vi "Lire Parameters.vi"(11 "Operation en entrée":refnum<class "Operation.lvclass">) -> (2 "Parameters":T1 {"Currency" items=["Euro", "Dollar", "Yen", "RIM", "CHF"]}, 3 "Operation en sortie":refnum<class "Operation.lvclass">)   [LabVIEW 2012, in "Operation.lvclass"]
uses:
  Operation.lvclass
  Operation Parameters.ctl
  Operation Type Enum.ctl
  controls/Currencies.ctl
  Operation.lvclass/Operation.ctl
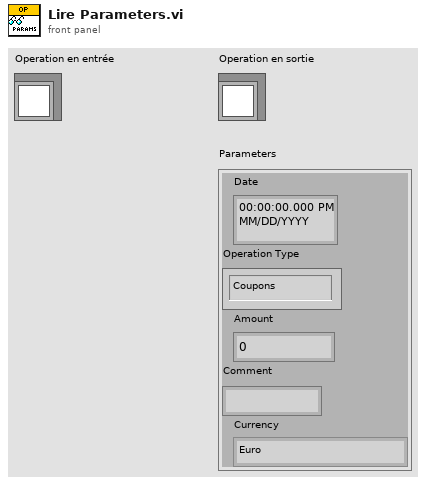
[diagram p1: front panel]
types:
  T1 = typedef "Operation Parameters.ctl" = cluster{"Date":timestamp, "Operation Type":T2, "Amount":dbl, "Comment":string, "Currency":T3}
  T2 = typedef "Operation Type Enum.ctl" = enum16{"Coupons", "Dépot", "Retrait", "Intérêts", "Taxe"}
  T3 = typedef "Currencies.ctl" = u16
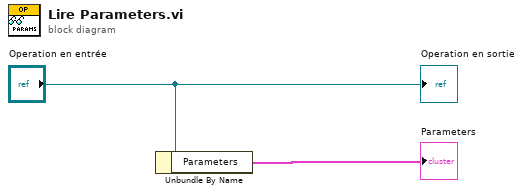
[diagram p0: block diagram]
diagram:
  n1 = Unbundle By Name("Operation en entrée") -> ("Parameters"=→"Parameters":T1)
  "Operation en sortie" <- "Operation en entrée"
